vi "Sequence File Reader.vi"(8 "error in":errorcluster, 11 "Select Sequencer File*":path) -> (0 "error out":errorcluster, 1 "AO":T1(array[cluster]), 2 "DO":T2(array[cluster]), 3 "all rows":string[][](array[string]))   [LabVIEW 2022 SP3]
uses:
  <vilib>/Utility/file.llb/Read Delimited Spreadsheet (string).vi
panel:
  # "e"
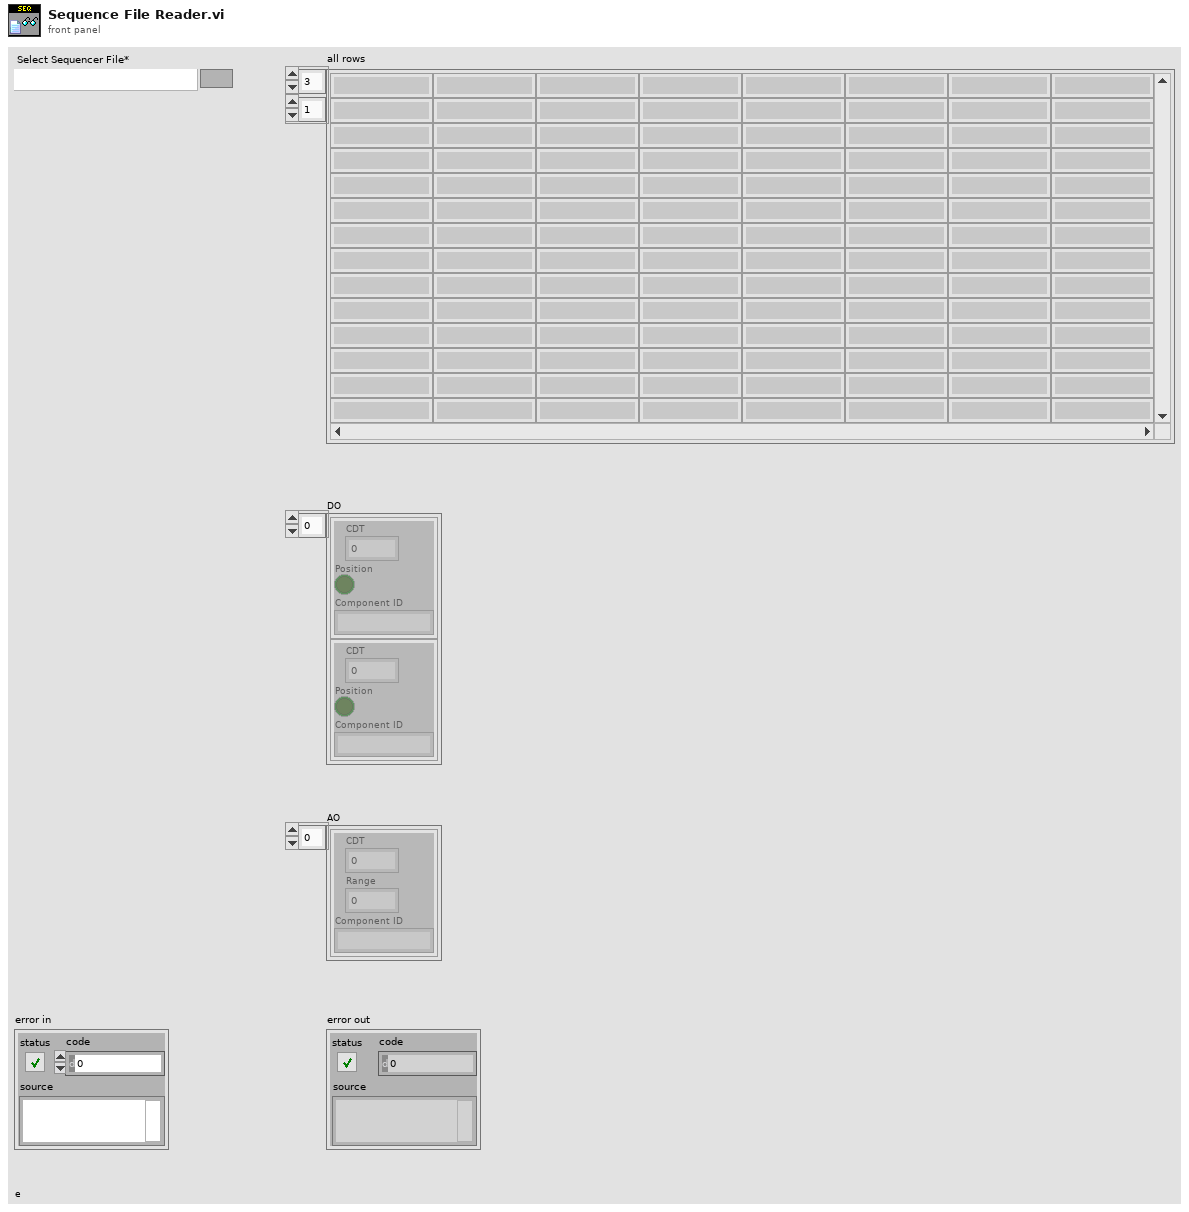
[diagram p1: front panel]
types:
  T1 = cluster{"CDT":dbl, "Range":dbl, "Component ID":string}[]
  T2 = cluster{"CDT":dbl, "Position":bool, "Component ID":string}[]
  T3 = cluster{"Sr. No.":string, "Time CDT":string, "Component ID":string, "Data Type":string, "Range/Position":string}
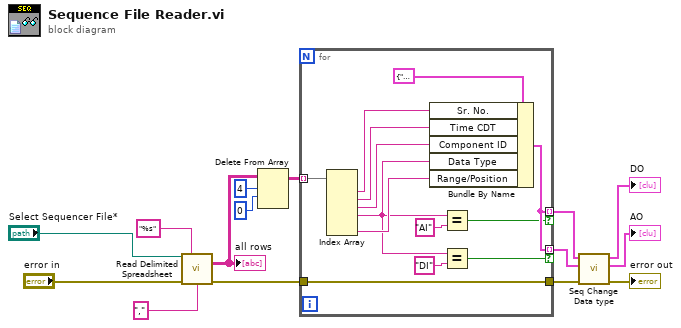
[diagram p0: block diagram]
diagram:
  n1 = call-poly <vilib>:"Read Delimited Spreadsheet.vi"("file path (dialog if empty)"="Select Sequencer File*", "format (%s)"="%s", "error in (no error)"="error in", "delimiter (\\t)"="," ("delimiter (\\t)")) -> ("all rows"=w10:string[][], "error out"=w8:errorcluster)  [unwired: 6 in, 4 out]
  "all rows" <- w10
  n2 = Delete From Array(array=w10, length=4, index (row)=0) -> (array with subset deleted=w11:string[][])  [unwired: 1 in, 1 out]
  n3 = for {
    tunnel: w11 -> [w28] mode=indexing
    tunnel: [w17] -> w4 mode=indexing if=w18
    tunnel: w8 -> [w23]
    tunnel: [w23] -> w2
    tunnel: [w17] -> w3 mode=indexing if=w16
    n4 = Index Array(array=w28) -> (element #1=w27:string, element #2=w26:string, element #3=w25:string, element #4=w19:string, element #6=w24:string)  [unwired: 6 in, 1 out]
    n5 = Bundle By Name(cluster=T3 {"Sr. No."="", "Time CDT"="", "Component ID"="", "Data Type"="", "Range/Position"=""} ("output cluster"), "Sr. No."=w27, "Time CDT"=w26, "Component ID"=w25, "Data Type"=w19, "Range/Position"=w24) -> (w17:T3)
    n6 = Equal?(x=w19, y="AI") -> (x = y?=w16:bool)
    n7 = Equal?(x=w19, y="DI") -> (x = y?=w18:bool)
  }
  n8 = call "Seq Change Data type.vi"("Error in"=w2, "DO Seq in"=w4, "AO Seq in"=w3) -> ("Error out"=→"error out":errorcluster, "AO"=→"AO":T1, "DO"=→"DO":T2)  [unwired: 6 in]
